vi "Actor Core.vi"(8 "error in":errorcluster, 11 "tWorkerController in":refnum<class "tWorkerController.lvclass">) -> (0 "error out":errorcluster, 3 "Actor out":refnum<class "Actor.lvclass">)   [LabVIEW 2013, in "tWorkerController.lvlib" / "tWorkerController.lvclass"]
doc: "(<B>Filename</B>: Actor Framework.lvlib:Actor.lvclass:Actor Core.vi)\n\nReceives messages to the actor, reacts to them, and initiates any error handling that may shut the actor down.\n\nDescendant classes may override this VI to append parallel tasks for the actor to complete while it handles messages. Overrides use the Call Parent Method node."
uses:
  tWorkerController.lvclass
  <vilib>/ActorFramework/Actor/Actor.lvclass
  tWorkerController.lvclass/tWorkerController.ctl
  <vilib>/ActorFramework/Actor/Actor.lvclass/Actor.ctl
  <vilib>/ActorFramework/Message Enqueuer/Message Enqueuer.lvclass/Message Enqueuer.ctl
  LVAutomationListener/msgs/Log Event Msg/Log Event Msg.lvclass/Log Event Msg.ctl
  msgs/Register New Connection Msg/Register New Connection Msg.lvclass/Register New Connection Msg.ctl
  msgs/TCP Listener Stop Msg/TCP Listener Stop Msg.lvclass/TCP Listener Stop Msg.ctl
  <vilib>/ActorFramework/Message Enqueuer/Init from Existing Queue.vi
  <vilib>/ActorFramework/Message Enqueuer/Enqueue.vi
  <vilib>/ActorFramework/Message Priority Queue/Priority Enqueue.vi
  <vilib>/ActorFramework/Message Enqueuer/Message Enqueuer.lvclass
  LVAutomationListener/msgs/Log Event Msg/Log Event Msg.lvclass
  msgs/Register New Connection Msg/Register New Connection Msg.lvclass
  msgs/TCP Listener Stop Msg/TCP Listener Stop Msg.lvclass
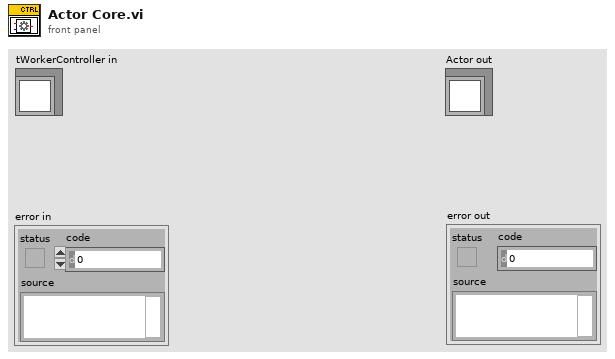
[diagram p1: front panel]
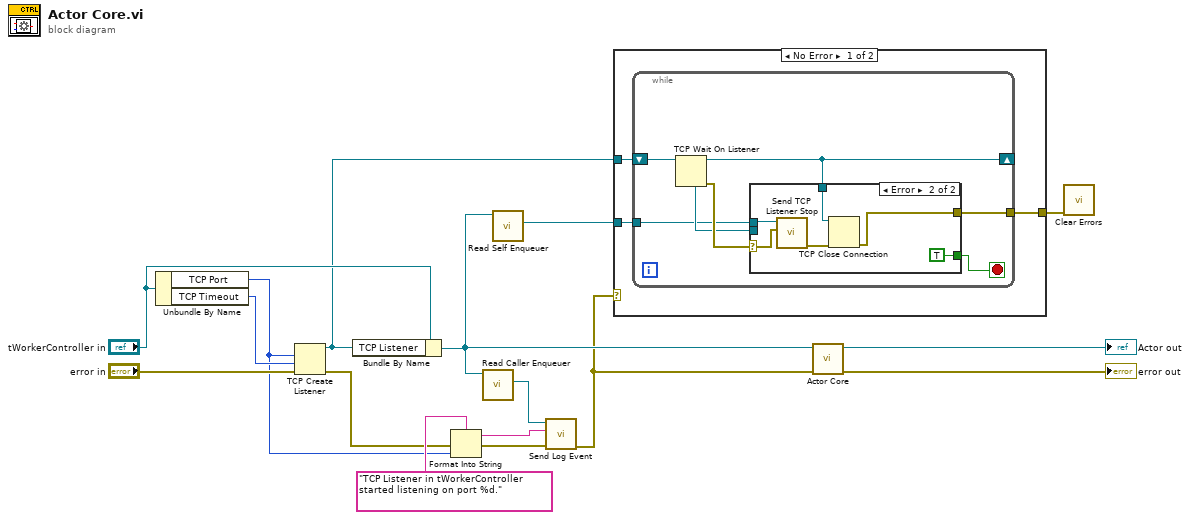
[diagram p0: block diagram]
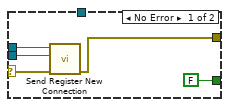
[diagram p2: hidden frame]
diagram:
  n1 = Unbundle By Name("tWorkerController in") -> ("TCP Port"=w1:u16, "TCP Timeout"=w12:i32)
  n2 = TCP Create Listener(8:"error in", 9:w12, 10:w1) -> (0:w4:errorcluster, 3:w10:refnum<k5>)  [unwired: 2 in, 1 out]
  n3 = Bundle By Name(cluster="tWorkerController in", "TCP Listener"=w10) -> (w7:refnum<class "tWorkerController.lvclass">)
  n4 = Format Into String(format string="TCP Listener in tWorkerController started listening on port %d.", error in=w4, w1) -> (resulting string=w2:string, error out=w3:errorcluster)  [unwired: 1 in]
  n5 = call <vilib>:"Read Caller Enqueuer.vi"("Actor"=w7) -> ("Caller Enqueuer"=w8:refnum<class "Message Enqueuer.lvclass">)  [unwired: 10 in]
  n6 = call <vilib>:"Read Self Enqueuer.vi"("Actor"=w7) -> ("Self Enqueuer"=w14:refnum<class "Message Enqueuer.lvclass">)  [unwired: 10 in]
  n7 = call "Send Log Event.vi"("error in (no error)"=w3, "Event Text"=w2, "Message Enqueuer"=w8) -> ("error out"=w6:errorcluster)  [unwired: 7 in, 1 out]
  n8 = case shown="No Error" w6 {
    selector: w6 -> [_ w38]
    tunnel: w14 -> [w19 _]
    tunnel: w10 -> [w18 _]
    tunnel: [w17 w38] -> w9
    frame No Error {
      n9 = while {
        tunnel: w19 -> [w23]
        shift-right: [w20] -> _
        shift-left: w18 -> [w26]
        tunnel: [w21] -> w17
        stop <- w22 stop-if-true
        n10 = TCP Wait On Listener(11:w26) -> (0:w25:errorcluster, 3:w20:refnum<k5>, 4:w24:refnum<k5>)  [unwired: 3 in, 2 out]
        n11 = case shown="Error" w25 {
          selector: w25 -> [w31 w35]
          tunnel: w24 -> [w29 _]
          tunnel: w23 -> [w30 w36]
          tunnel: [FALSE TRUE] -> w22
          tunnel: [w27 w32] -> w21
          tunnel: w20 -> [_ w33]
          frame No Error {
            n12 = call "Send Register New Connection.vi"("error in (no error)"=w31, "TCP Connection"=w29, "Message Enqueuer"=w30) -> ("error out"=w27:errorcluster)  [unwired: 7 in, 1 out]
          }
          frame Error {
            n13 = call "Send TCP Listener Stop.vi"("Listener Error"=w35, "Message Enqueuer"=w36) -> ("error out"=w34:errorcluster)  [unwired: 8 in, 1 out]
            n14 = TCP Close Connection(connection ID=w33, error in (no error)=w34) -> (error out=w32:errorcluster)  [unwired: 1 in, 1 out]
          }
        }
      }
    }
    frame Error {
    }
  }
  n15 = call-parent "Actor Core.vi"("error in"=w6, "Actor in"=w7) -> ("error out"=→"error out":errorcluster, "Actor out"=→"Actor out":refnum<class "Actor.lvclass">)  [unwired: 8 in]
  n16 = call <vilib>:"Clear Errors.vi"("error in (no error)"=w9) -> ()  [unwired: 6 in, 1 out]
